vi "mxwScript_API_XMLChainEndConnectDataToXML.vi"(8 "error in (no error)":errorcluster, 11 "connect in":T1={"connect?"=FALSE, "final label"="Test", "use index?"=FALSE, "connPaneIndex"=0, "area"=enum."TopLeft", "connection type"=enum."Recommended"}) -> (0 "error out":errorcluster, 3 "ConnectXML":string)   [LabVIEW 2020]
uses:
  codeGenAPISupport.llb/cgAPI_mxwScript_Wire_ChnCnnctStartEndData.ctl
  codeGenAPISupport.llb/cgAPI_mxwScript_ConnPaneArea.ctl
  codeGenAPISupport.llb/cgAPI_mxwScript_ConnPaneConnectionType.ctl
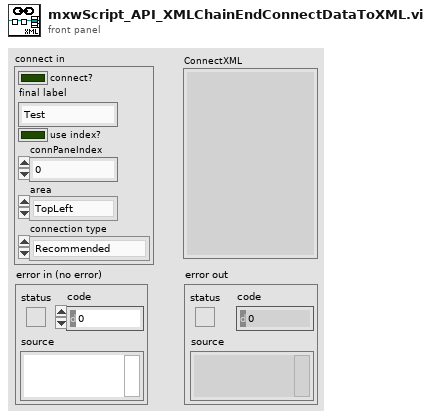
[diagram p1: front panel]
types:
  T1 = typedef "cgAPI_mxwScript_Wire_ChnCnnctStartEndData.ctl" = cluster{"connect?":bool, "final label":string, "use index?":bool, "connPaneIndex":i32, "area":T2, "connection type":T3}
  T2 = typedef "cgAPI_mxwScript_ConnPaneArea.ctl" = enum16{"TopLeft", "Top", "TopRight", "Right", "BottomRight", "Bottom", "BottomLeft", "Left"}
  T3 = typedef "cgAPI_mxwScript_ConnPaneConnectionType.ctl" = enum16{"Invalid Wire Rule", "Required", "Recommended", "Optional", "Dynamic Dispatch"}
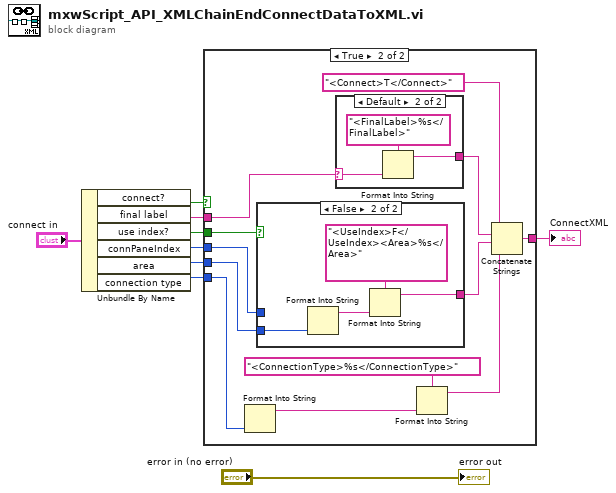
[diagram p0: block diagram]
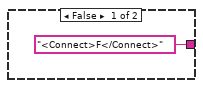
[diagram p2: hidden frame]
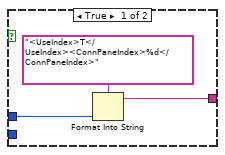
[diagram p3: hidden frame]
diagram:
  n1 = Unbundle By Name("connect in") -> ("connect?"=w3:bool, "final label"=w4:string, "use index?"=w8:bool, "connPaneIndex"=w7:i32, "area"=w6:T2, "connection type"=w5:T3)
  n2 = case shown="True" w3 {
    tunnel: ["<Connect>F</Connect>" w14] -> w9
    tunnel: w4 -> [_ w21]
    tunnel: w5 -> [_ w12]
    tunnel: w6 -> [_ w17]
    tunnel: w7 -> [_ w18]
    tunnel: w8 -> [_ w19]
    frame False {
    }
    frame True {
      n3 = Format Into String(w12) -> (resulting string=w11:string)  [unwired: 3 in, 1 out]
      n4 = case shown="False" w19 {
        tunnel: w18 -> [w24 _]
        tunnel: w17 -> [_ w27]
        tunnel: [w23 w28] -> w16
        frame True {
          n5 = Format Into String(format string="<UseIndex>T</UseIndex><ConnPaneIndex>%d</ConnPaneIndex>" ("string"), w24) -> (resulting string=w23:string)  [unwired: 2 in, 1 out]
        }
        frame False {
          n6 = Format Into String(w27) -> (resulting string=w26:string)  [unwired: 3 in, 1 out]
          n7 = Format Into String(format string="<UseIndex>F</UseIndex><Area>%s</Area>" ("string"), w26) -> (resulting string=w28:string)  [unwired: 2 in, 1 out]
        }
      }
      n8 = case shown="Default" w21 {
        selector: w21 -> [w30 w32]
        tunnel: [w30 w31] -> w20
        frame "" {
        }
        frame Default {
          n9 = Format Into String(format string="<FinalLabel>%s</FinalLabel>" ("string"), w32) -> (resulting string=w31:string)  [unwired: 2 in, 1 out]
        }
      }
      n10 = Format Into String(format string="<ConnectionType>%s</ConnectionType>", w11) -> (resulting string=w15:string)  [unwired: 2 in, 1 out]
      n11 = Concatenate Strings("<Connect>T</Connect>", w20, w16, w15) -> (w14:string)
    }
  }
  "ConnectXML" <- w9
  "error out" <- "error in (no error)"
